vi "toUCharScalar.vi"(2 "value_in":u8[](array[numeric]), 3 "dim_y":i32, 4 "dim_x":i32) -> (0 "setpoint":u8, 1 "value_out":u8)   [LabVIEW 2014, in "tango.lvlib"]
uses:
  tango.lvlib
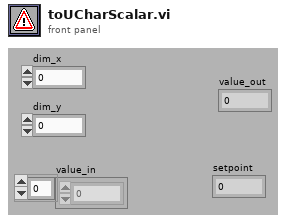
[diagram p1: front panel]
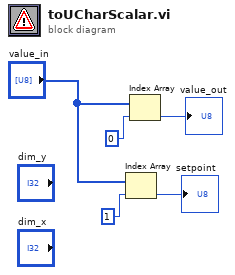
[diagram p0: block diagram]
diagram:
  n1 = Index Array(array="value_in", index=1 ("indice")) -> (element=→"setpoint":u8)
  n2 = Index Array(array="value_in", index=0 ("indice")) -> (element=→"value_out":u8)
